vi "Close Report.vi"(2 "error in (no error)":errorcluster, 3 "Save Changes?":bool, 4 "Report Ref In":T1) -> (0 "error out":errorcluster, 1 "Report Ref Out":T1)   [LabVIEW 2013, in "XCel Report Engine.lvlib"]
doc: "Closes an open XCelReportEngine report session and releases its associated resources.\n\nWhen Save Changes is TRUE, the workbook is saved to the output path specified by New Report.vi before the session is closed. When FALSE, any changes made since the last explicit save are discarded.\n\nAfter this VI executes successfully, Report Ref is no longer valid and must not be used by subsequent report operations.\n\nCall this VI for every report session created by New Report.vi, including error-handling paths."
uses:
  XCel Report Engine.lvlib
  Controls/Report Ref.ctl
  C:/Users/m.santucci/Documents/ChatGPT/LV_REPORT_ENGINE/LV/DotNet/XCelReportEngine.dll
  LV/DotNet/XCelReportEngine.dll
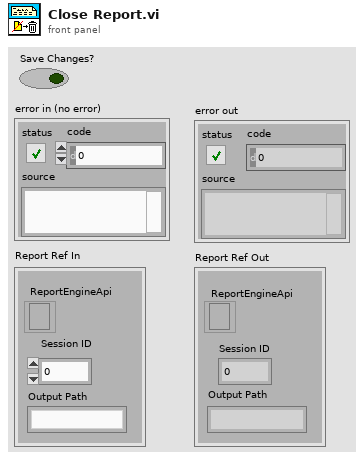
[diagram p1: front panel]
types:
  T1 = typedef "XCel Report Engine.lvlib/Report Ref.ctl" = cluster{"Session ID":i32, "Output Path":string, "ReportEngineApi":refnum<k24>}
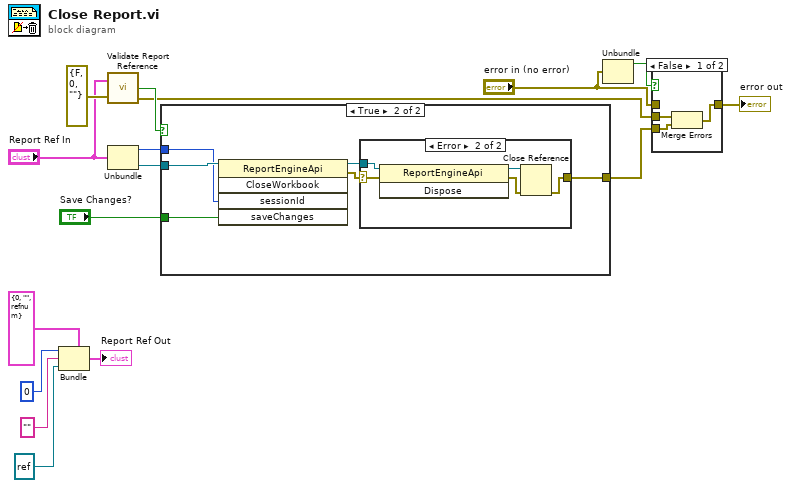
[diagram p0: block diagram]
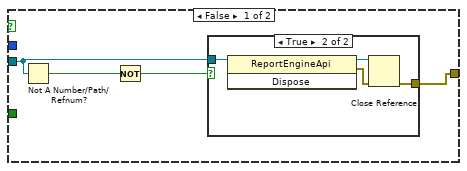
[diagram p3: hidden frame]
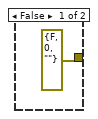
[diagram p4: hidden frame]
diagram:
  n1 = Bundle(cluster=T1 {"Session ID"=0, "Output Path"="", "ReportEngineApi"=refnum} ("Report Ref"), "Session ID"=0, "Output Path"="", "ReportEngineApi"=refnum<k24> refnum) -> (→"Report Ref Out":T1)
  n2 = call "Validate Report Reference.vi"("Report Ref In"="Report Ref In", "error in (no error)"=errorcluster {"status"=FALSE, "code"=0, "source"=""}) -> ("Valid"=w11:bool, "error out"=w2:errorcluster)  [unwired: 1 out]
  n3 = Unbundle("Report Ref In") -> ("Session ID"=w15:i32, "ReportEngineApi"=w16:refnum<k24>)  [unwired: 1 out]
  n4 = case shown="True" w11 {
    tunnel: w16 -> [w18 w31]
    tunnel: w15 -> [_ w30]
    tunnel: "Save Changes?" -> [_ w29]
    tunnel: [w17 w26] -> w1
    frame False {
      n5 = Not A Number/Path/Refnum?(number/path/refnum=w18) -> (NaN/Path/Refnum?=w20:bool)
      n6 = Not(x=w20) -> (.not. x?=w19:bool)
      n7 = case shown="True" w19 {
        tunnel: w18 -> [_ w24]
        tunnel: [errorcluster {"status"=FALSE, "code"=0, "source"=""} ("error out") w23] -> w17
        frame False {
        }
        frame True {
          n8 = invoke class="ReportEngineApi" method="Dispose"(reference=w24) -> (reference out=w22:refnum<k24>, error out=w25:errorcluster)  [unwired: 2 in, 1 out]
          n9 = Close Reference(reference=w22, error in (no error)=w25) -> (error out=w23:errorcluster)
        }
      }
    }
    frame True {
      n10 = invoke class="ReportEngineApi" method="CloseWorkbook"(reference=w31, "sessionId"=w30, "saveChanges"=w29) -> (reference out=w28:refnum<k24>, error out=w27:errorcluster)  [unwired: 2 in, 3 out]
      n11 = case shown="Error" w27 {
        selector: w27 -> [w32 w35]
        tunnel: w28 -> [_ w37]
        tunnel: [w32 w33] -> w26
        frame No Error {
        }
        frame Error {
          n12 = invoke class="ReportEngineApi" method="Dispose"(reference=w37, error in=w35) -> (reference out=w36:refnum<k24>, error out=w34:errorcluster)  [unwired: 1 in, 1 out]
          n13 = Close Reference(reference=w36, error in (no error)=w34) -> (error out=w33:errorcluster)
        }
      }
    }
  }
  n14 = Unbundle("error in (no error)") -> ("status"=w10:bool)  [unwired: 2 out]
  n15 = case shown="False" w10 {
    tunnel: "error in (no error)" -> [_ w41]
    tunnel: [w40 w41] -> w8
    tunnel: w2 -> [w39 _]
    tunnel: w1 -> [w38 _]
    frame False {
      n16 = Merge Errors(w39, w38) -> (w40:errorcluster)
    }
    frame True {
    }
  }
  "error out" <- w8
